vi "Database.AddComponent.vi"(7 "Idx":i32, 8 "error in":errorcluster, 10 "Product Component":T1, 11 "Data in":T2) -> (0 "error out":errorcluster, 1 "ExportTS":timestamp, 3 "Data out":T2)   [LabVIEW 2016]
uses:
  Database.Data.ctl
  Database.Data.Status.ctl
  Database.Data.Sets.ctl
  ProdaNG/Controls/ProdaNG.ProductComponent.ctl
  Tools/Translator/Translator.Message.ctl
  Tools/EventLog/EventLog.EventSource.ctl
  Tools/EventLog/EventLog.New(array).vi
  Global/ApplicationGlobal.vi
  Tools/EventLog/EventLog.Buffer.vi
  Tools/EventLog/EventLog.File.ReadWrite.vi
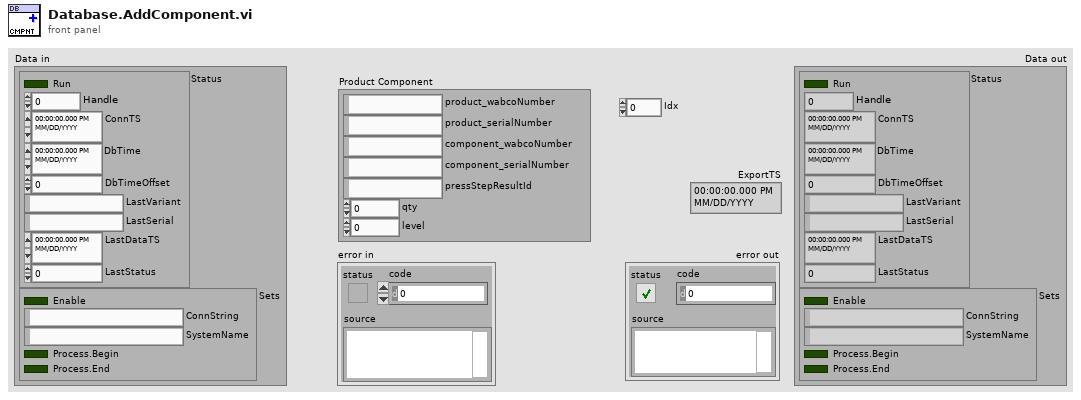
[diagram p1: front panel]
types:
  T1 = typedef "ProdaNG.ProductComponent.ctl" = cluster{"product_wabcoNumber":string, "product_serialNumber":string, "component_wabcoNumber":string, "component_serialNumber":string, "pressStepResultId":string, "qty":i32, "level":i32}
  T2 = typedef "Database.Data.ctl" = cluster{"Status":T3, "Sets":T4}
  T3 = typedef "Database.Data.Status.ctl" = cluster{"Run":bool, "Handle":i32, "ConnTS":timestamp, "DbTime":timestamp, "DbTimeOffset":dbl, "LastVariant":string, "LastSerial":string, "LastDataTS":timestamp, "LastStatus":i32}
  T4 = typedef "Database.Data.Sets.ctl" = cluster{"Enable":bool, "ConnString":string, "SystemName":string, "Process.Begin":bool, "Process.End":bool}
  T5 = typedef "EventLog.EventSource.ctl" = enum16{"All", "Gui", "Cache", "PLC1", "PLC2", "PLC3", "DB", "DB01", "DB02", "DB03", "DB04", "DB05", "DB06", "DB07", "DB08", "DB09", "DB10", "DB11", "DB12", "DB13", "DB14", "DB15", "DB16"}
  T6 = typedef "Translator.Message.ctl" = enum16{"-", "Event confirmed", "Log out", "Log in", "Shutdown", "Cancel", "Start", "Continue", "Stop", "On", "Off", "OK", "NOK", "NOK %s", "This", "Prev", "Home", "Work", "In progress...", "Missing", "Empty", "Hardware failure", "Initial", "Error %d >> %s", "Error %d >> %s >> %s", "Starting %s", "Quitting %s", "Configured", "Initializing", "Quitting", "Loading", "Running %s", "Stopped", "Summary", "Do you want to continue?", "Do you want to exit?", "Log out?", "System", "All", "IDLE", "Translating...%s", "Not found", "Alarm %s", "Run", "Skip", "Abort", "Repeat", "Please wait...", "Database disconnected", "Login to database successful", "Login to database failed: %d; %s", "Get process step data for %s", "Changeover off", "Changeover into %s", "Product %s | %s found in cache with status %d at previous station", "Product %s | %s found in database with status %d at previous station", "Product %s | %s not found in cache at previous station", "Product %s | %s not found in database at previous station", "Product %s | %s found in cache with status %d at this station (%d repetion)", "Product %s | %s found in database with status %d at this station (%d repetition)", "Product %s | %s not found in cache at this station", "Product %s | %s not found in database at this station", "Product %s | %s found in cache for component %s | %s", "Product %s | %s found in database for component %s | %s", "Product not found in cache for component %s | %s", "Product not found in database for component %s | %s", "Product %s | %s connected with component %s | %s (cache)", "Product %s | %s connected with component %s | %s (database)", "New data for %s | %s (cache)", "New data for %s | %s (database)", "File %s moved (cache)", "File %s deleted (cache)", "Msg %d >> %s", "PLC LifeBit Failure", "Reconnecting DB", "Reconnecting PLC", "Free disk space is below 1GB - contact technician"}
  T7 = typedef "Database.Data.Variant.Sets.ctl" = cluster{"PrevStations":string[], "ThisStations":string[]}
  T8 = typedef "ProdaNG.Identification.ctl" = cluster{"processId":i32, "systemId":i32, "processStepId":i32, "wabcoPartId":i32}
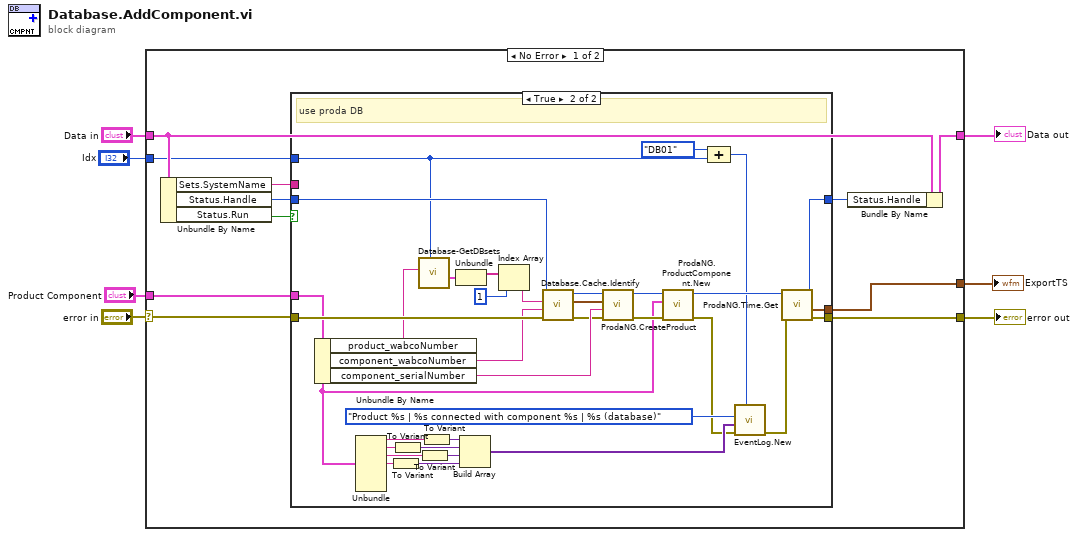
[diagram p0: block diagram]
diagram:
  n1 = case shown="No Error" "error in" {
    selector: "error in" -> [w18 w56]
    tunnel: [w12 w56] -> w7
    tunnel: "Data in" -> [w16 w55]
    tunnel: [w15 w55] -> w4
    tunnel: "Product Component" -> [w11 _]
    tunnel: [w9 _] -> w2
    tunnel: "Idx" -> [w8 _]
    frame No Error {
      n2 = Unbundle By Name(w16) -> ("Sets.SystemName"=w10:string, "Status.Handle"=w17:i32, "Status.Run"=w13:bool)
      n3 = case shown="True" w13 {
        tunnel: w18 -> [w20 w44]
        tunnel: w17 -> [w19 w43]
        tunnel: [w19 w48] -> w14
        tunnel: [w20 w53] -> w12
        tunnel: w11 -> [_ w34]
        tunnel: w10 -> [_ _]
        tunnel: [_ w52] -> w9
        tunnel: w8 -> [_ w26]
        frame False {
        }
        frame True {
          # "use proda DB"
          n4 = Unbundle By Name(w34) -> ("product_wabcoNumber"=w21:string, "component_wabcoNumber"=w27:string, "component_serialNumber"=w54:string)
          n5 = Unbundle(w34) -> ("product_wabcoNumber"=w33:string, "product_serialNumber"=w32:string, "component_wabcoNumber"=w31:string, "component_serialNumber"=w30:string)  [unwired: 3 out]
          n6 = To Variant(anything=w30) -> (Variant=w39:variant)
          n7 = To Variant(anything=w32) -> (Variant=w42:variant)
          n8 = call "Database-GetDBsets.vi"("Idx"=w26, "Variant"=w21) -> ("Variant Sets"=w25:T7)  [unwired: 5 in, 4 out]
          n9 = To Variant(anything=w31) -> (Variant=w40:variant)
          n10 = To Variant(anything=w33) -> (Variant=w41:variant)
          n11 = Unbundle(w25) -> ("PrevStations"=w23:string[])  [unwired: 1 out]
          n12 = Build Array(w41, w42, w40, w39) -> (w38:variant[])
          n13 = Index Array(array=w23, index=1) -> (element=w22:string)
          n14 = call "Database.Cache.Identify.vi"("error in (no error)"=w44, "Variant"=w27, "SystemName"=w22, "DB Handle in"=w43) -> ("error out"=w47:errorcluster, "SytemID"=w46:T8, "DB Handle out"=w45:i32)  [unwired: 5 in]
          n15 = call "ProdaNG.CreateProduct.vi"("error in (no error)"=w47, "serialNumber"=w54, "ID"=w46, "dbHandle"=w45) -> ("error out"=w51:errorcluster, "dbHandle out"=w50:i32)  [unwired: 5 in, 1 out]
          n16 = call "ProdaNG.ProductComponent.New.vi"("error in (no error)"=w51, "Product Component"=w34, "dbHandle"=w50) -> ("error out"=w28:errorcluster, "dbHandle"=w49:i32)  [unwired: 7 in]
          n17 = Compound Arithmetic op=ADD(EventLog.EventSource."DB01" ("Source (All)"), w26) -> (w35:i32)
          n18 = call-poly "EventLog.New.vi"("Source (All)"=w35, "error in (no error)"=w28, "Arguments"=w38, "Message (-)"=Translator.Message."Product %s | %s connected with component %s | %s (database)") -> ("error out"=w29:errorcluster)  [unwired: 6 in, 1 out]
          n19 = call "ProdaNG.Time.Get.vi"("error in"=w29, "dbHandleIn"=w49) -> ("error out"=w53:errorcluster, "time"=w52:timestamp, "dbHandle"=w48:i32)  [unwired: 5 in, 1 out]
        }
      }
      n20 = Bundle By Name(cluster=w16, "Status.Handle"=w14) -> (w15:T2)
    }
    frame Error {
    }
  }
  "error out" <- w7
  "Data out" <- w4
  "ExportTS" <- w2
